vi "WW_GatherSpinParameter_V2.vi"(11 "路径":path) -> (0 "strFinishStepIndex":T1, 1 "strFinalSpinStepIndex":T2, 2 "strProgressStateIndex":T3, 3 "strPowerStateIndex":T5, 4 "EXCEL读取":string[][](array[string]), 5 "ms32ArrayLength":i32, 6 "strInitProgressStepIndex":T4)   [LabVIEW 2011]
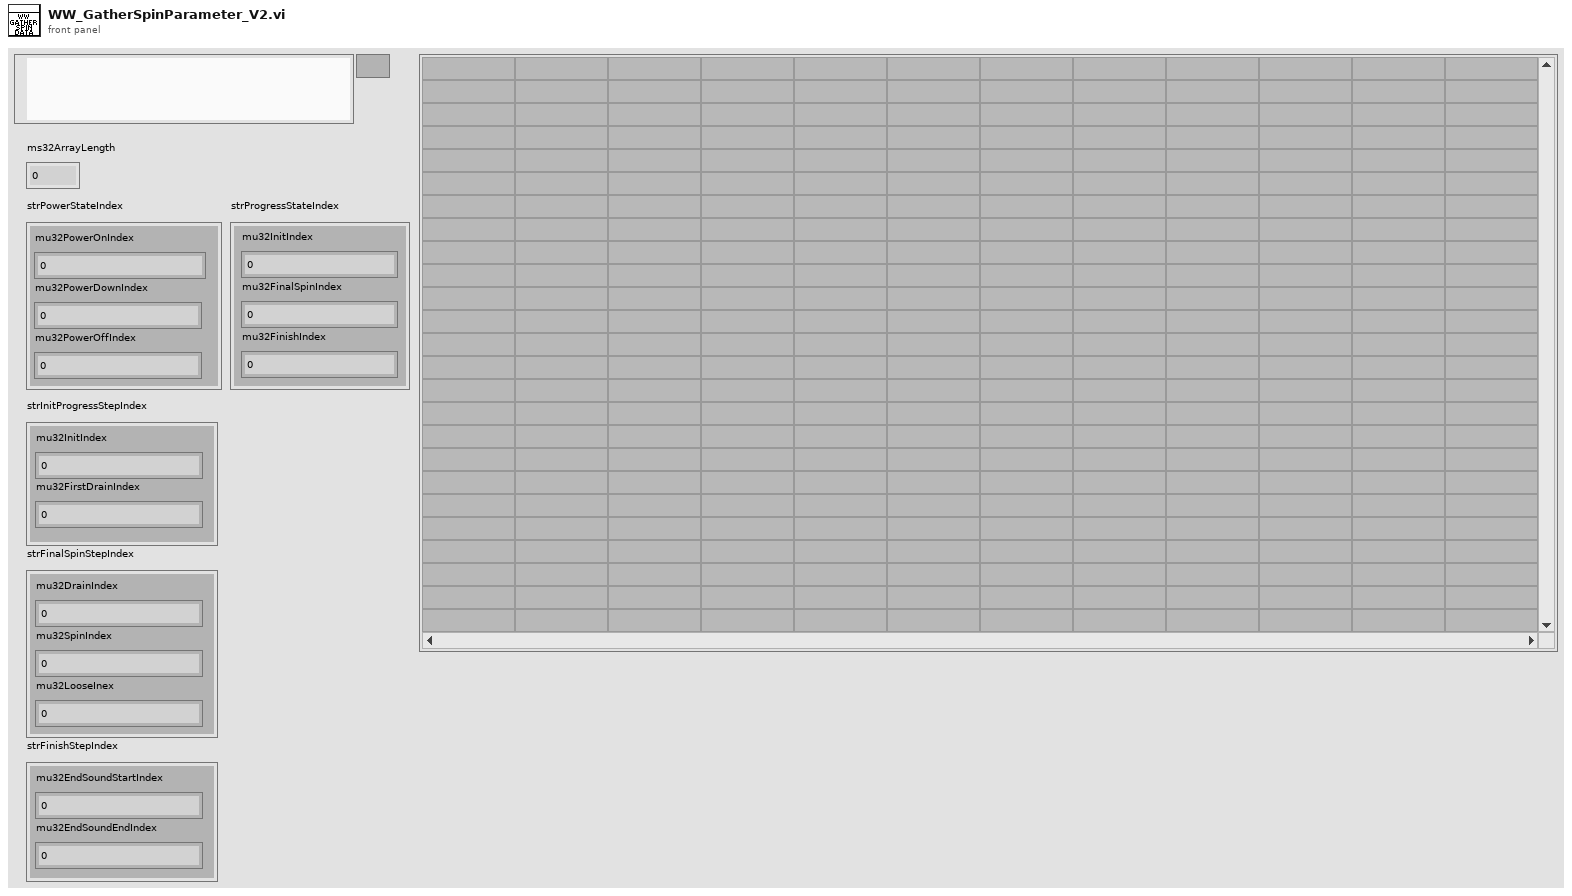
[diagram p1: front panel]
types:
  T1 = cluster{"mu32EndSoundStartIndex":u32, "mu32EndSoundEndIndex":u32}
  T2 = cluster{"mu32DrainIndex":u32, "mu32SpinIndex":u32, "mu32LooseInex":u32}
  T3 = cluster{"mu32InitIndex":u32, "mu32FinalSpinIndex":u32, "mu32FinishIndex":u32}
  T4 = cluster{"mu32InitIndex":u32, "mu32FirstDrainIndex":u32}
  T5 = cluster{"mu32PowerOnIndex":u32, "mu32PowerDownIndex":u32, "mu32PowerOffIndex":u32}
  T6 = enum16{"RealTime", "WaterLevel", "WaterTemp", "AirTemp", "IPMTemp", "MotorActualRPM", "MotorTargetRPM", "FanActualRPM", "MemsSensorA", "MemsSensorB", "MemsSensorC", "WaterThermistorADC", "TouchSensor", "LeakageSensor", "DCLink", "IsDoorOpen", "IsTimeShort", "Progress", "Step", "TotalRemainTime", "StepRemainTime", "WeightSensingLowData", "WeightSensingResult", "ColdValve", "HotValve", "PreValve", "WaterShotValve", "BleachValve", "DryValve", "SteamValve", "SoftenerValve", "FilterValve", "IsDoorLocked", "SSRCommon", "MainRelay", "ACTUATOR2", "WaterDrainer", "CirculationPump", "WaterHeater", "DryHeater", "SteamHeater", "MotorDriveDirection", "IsDoubleDoorOpen", "IsDoubleDoorLock", "RunStateID", "PowerStateID", "SoundID", "ErrorCode", "OptionData", "MainVersion", "SUBVersion", "InverterVersion"}
  T7 = enum16{"POWER_STATE_POWER_OFF", "POWER_STATE_POWER_UP_INIT", "POWER_STATE_POWER_UP_START", "POWER_STATE_POWER_UP_DONE", "POWER_STATE_POWER_ON", "POWER_STATE_POWER_DOWN", "POWER_STATE_POWER_OFF_FOR_OTN", "POWER_STATE_POWER_SLEEP_MODE"}
  T8 = enum16{"PROGRESS_INITIAL", "PROGRESS_RESERVE", "PROGRESS_PREWASH", "PROGRESS_WASH", "PROGRESS_RINSE", "PROGRESS_FINALSPIN", "PROGRESS_DRY", "PROGRESS_AIRWASH", "PROGRESS_FINISH", "PROGRESS_END", "PROGRESS_MAX"}
  T9 = enum16{"INIT_PROGRESS_INIT", "INIT_PROGRESS_FIRST_DRAIN_INITIAL", "INIT_PROGRESS_FIRST_DRAIN"}
  T10 = enum16{"FINALSPIN_INIT", "FINALSPIN_DRAIN", "FINALSPIN_SUDS_REDUCTION", "FINALSPIN_SPIN", "FINALSPIN_LOOSE", "FINALSPIN_END"}
  T11 = enum16{"FINISH_STEPORDER_COUNT_INFORMATION_SAVE", "FINISH_STEPORDER_ENDSOUND_PLAY", "FINISH_STEPORDER_UNLOCK_CHECK", "FINISH_STEPORDER_AGING_WAITTIME_CHECK", "FINISH_STEPORDER_AGING_WAITTING", "FINISH_STEPORDER_NOMAL_WAITTING", "FINISH_STEPORDER_DRUMLIGHT_CHECK", "FINISH_STEPORDER_CHECK_MOTOR_STOP", "FINISH_STEPORDER_CHILDLOCK_WAITTING", "FINISH_STEPORDER_CLOSE"}
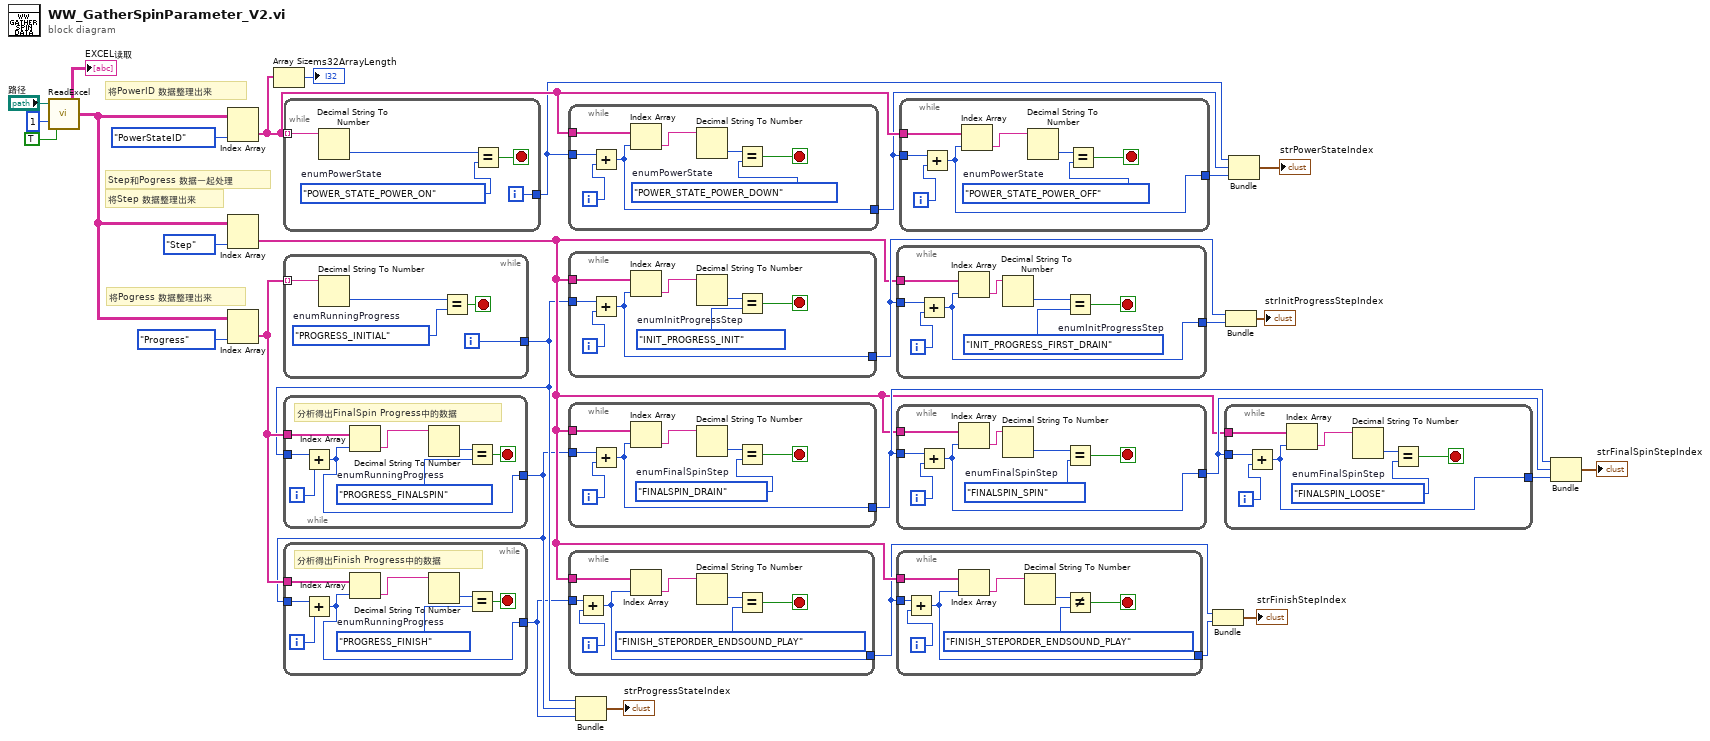
[diagram p0: block diagram]
diagram:
  # "Step和Pogress 数据一起处理"
  # "将Step 数据整理出来"
  # "将Pogress 数据整理出来"
  # "将PowerID 数据整理出来"
  n1 = call "ReadExcel.vi"("读出文本"=TRUE, "导出sheet位号"=i8 1, "路径"="路径") -> ("EXCEL读取"=w15:string[][])
  "EXCEL读取" <- w15
  n2 = Index Array(array=w15, index (col)=T6."PowerStateID" ("WW_ParameterData")) -> (element=w24:string[])  [unwired: 1 in]
  n3 = Index Array(array=w15, index (col)=T6."Step" ("WW_ParameterData")) -> (element=w8:string[])  [unwired: 1 in]
  n4 = Index Array(array=w15, index (col)=T6."Progress" ("WW_ParameterData")) -> (element=w9:string[])  [unwired: 1 in]
  n5 = Array Size(array=w24) -> (size(s)=→"ms32ArrayLength":i32)
  n6 = while {
    tunnel: w24 -> [w34] mode=indexing
    tunnel: [w30] -> w23
    i -> [w30]
    stop <- w31 stop-if-true
    w32 = T7."POWER_STATE_POWER_ON"  # enumPowerState
    n7 = Decimal String To Number(string=w34) -> (number=w33:i32)  [unwired: 2 in, 1 out]
    n8 = Equal?(x=w33, y=w32) -> (x = y?=w31:bool)
  }
  n9 = while {
    tunnel: w9 -> [w39] mode=indexing
    tunnel: [w36] -> w4
    i -> [w36]
    stop <- w37 stop-if-true
    w35 = T8."PROGRESS_INITIAL"  # enumRunningProgress
    n10 = Decimal String To Number(string=w39) -> (number=w38:i32)  [unwired: 2 in, 1 out]
    n11 = Equal?(x=w38, y=w35) -> (x = y?=w37:bool)
  }
  n12 = while {
    tunnel: w9 -> [w42]
    tunnel: w4 -> [w43]
    tunnel: [w40] -> w3
    i -> [w44]
    stop <- w46 stop-if-true
    w45 = T8."PROGRESS_FINALSPIN"  # enumRunningProgress
    # "分析得出FinalSpin Progress中的数据"
    n13 = Add(x=w43, y=w44) -> (x+y=w40:i32)
    n14 = Index Array(array=w42, index=w40) -> (element=w41:string)
    n15 = Decimal String To Number(string=w41) -> (number=w47:i32)  [unwired: 2 in, 1 out]
    n16 = Equal?(x=w47, y=w45) -> (x = y?=w46:bool)
  }
  n17 = while {
    tunnel: w9 -> [w50]
    tunnel: w3 -> [w51]
    tunnel: [w48] -> w2
    i -> [w52]
    stop <- w54 stop-if-true
    w53 = T8."PROGRESS_FINISH"  # enumRunningProgress
    # "分析得出Finish Progress中的数据"
    n18 = Add(x=w51, y=w52) -> (x+y=w48:i32)
    n19 = Index Array(array=w50, index=w48) -> (element=w49:string)
    n20 = Decimal String To Number(string=w49) -> (number=w55:i32)  [unwired: 2 in, 1 out]
    n21 = Equal?(x=w55, y=w53) -> (x = y?=w54:bool)
  }
  n22 = while {
    tunnel: w24 -> [w58]
    tunnel: w23 -> [w59]
    tunnel: [w56] -> w22
    i -> [w60]
    stop <- w61 stop-if-true
    w62 = T7."POWER_STATE_POWER_DOWN"  # enumPowerState
    n23 = Add(x=w59, y=w60) -> (x+y=w56:i32)
    n24 = Index Array(array=w58, index=w56) -> (element=w57:string)
    n25 = Decimal String To Number(string=w57) -> (number=w63:i32)  [unwired: 2 in, 1 out]
    n26 = Equal?(x=w63, y=w62) -> (x = y?=w61:bool)
  }
  n27 = while {
    tunnel: w8 -> [w67]
    tunnel: w4 -> [w68]
    tunnel: [w65] -> w18
    i -> [w69]
    stop <- w70 stop-if-true
    w64 = T9."INIT_PROGRESS_INIT"  # enumInitProgressStep
    n28 = Add(x=w68, y=w69) -> (x+y=w65:i32)
    n29 = Index Array(array=w67, index=w65) -> (element=w66:string)
    n30 = Decimal String To Number(string=w66) -> (number=w71:i32)  [unwired: 2 in, 1 out]
    n31 = Equal?(x=w71, y=w64) -> (x = y?=w70:bool)
  }
  n32 = while {
    tunnel: w8 -> [w75]
    tunnel: w3 -> [w76]
    tunnel: [w73] -> w13
    i -> [w77]
    stop <- w78 stop-if-true
    w72 = T10."FINALSPIN_DRAIN"  # enumFinalSpinStep
    n33 = Add(x=w76, y=w77) -> (x+y=w73:i32)
    n34 = Index Array(array=w75, index=w73) -> (element=w74:string)
    n35 = Decimal String To Number(string=w74) -> (number=w79:i32)  [unwired: 2 in, 1 out]
    n36 = Equal?(x=w79, y=w72) -> (x = y?=w78:bool)
  }
  n37 = while {
    tunnel: w8 -> [w83]
    tunnel: w2 -> [w84]
    tunnel: [w81] -> w7
    i -> [w85]
    stop <- w86 stop-if-true
    n38 = Add(x=w84, y=w85) -> (x+y=w81:i32)
    n39 = Index Array(array=w83, index=w81) -> (element=w82:string)
    n40 = Decimal String To Number(string=w82) -> (number=w87:i32)  [unwired: 2 in, 1 out]
    n41 = Equal?(x=w87, y=T11."FINISH_STEPORDER_ENDSOUND_PLAY" ("enumFinishStep")) -> (x = y?=w86:bool)
  }
  n42 = Bundle(w4, w3, w2) -> (→"strProgressStateIndex":cluster{i32, i32, i32})  [unwired: 1 in]
  n43 = while {
    tunnel: w8 -> [w91]
    tunnel: w18 -> [w92]
    tunnel: [w89] -> w17
    i -> [w93]
    stop <- w94 stop-if-true
    w88 = T9."INIT_PROGRESS_FIRST_DRAIN"  # enumInitProgressStep
    n44 = Add(x=w92, y=w93) -> (x+y=w89:i32)
    n45 = Index Array(array=w91, index=w89) -> (element=w90:string)
    n46 = Decimal String To Number(string=w90) -> (number=w95:i32)  [unwired: 2 in, 1 out]
    n47 = Equal?(x=w95, y=w88) -> (x = y?=w94:bool)
  }
  n48 = while {
    tunnel: w8 -> [w99]
    tunnel: w13 -> [w100]
    tunnel: [w97] -> w12
    i -> [w101]
    stop <- w102 stop-if-true
    w96 = T10."FINALSPIN_SPIN"  # enumFinalSpinStep
    n49 = Add(x=w100, y=w101) -> (x+y=w97:i32)
    n50 = Index Array(array=w99, index=w97) -> (element=w98:string)
    n51 = Decimal String To Number(string=w98) -> (number=w103:i32)  [unwired: 2 in, 1 out]
    n52 = Equal?(x=w103, y=w96) -> (x = y?=w102:bool)
  }
  n53 = while {
    tunnel: w8 -> [w107]
    tunnel: w7 -> [w108]
    tunnel: [w105] -> w6
    i -> [w109]
    stop <- w110 stop-if-true
    n54 = Add(x=w108, y=w109) -> (x+y=w105:i32)
    n55 = Index Array(array=w107, index=w105) -> (element=w106:string)
    n56 = Decimal String To Number(string=w106) -> (number=w111:i32)  [unwired: 2 in, 1 out]
    n57 = Not Equal?(x=w111, y=T11."FINISH_STEPORDER_ENDSOUND_PLAY" ("enumFinishStep")) -> (x != y?=w110:bool)
  }
  n58 = while {
    tunnel: w24 -> [w114]
    tunnel: w22 -> [w115]
    tunnel: [w112] -> w21
    i -> [w116]
    stop <- w117 stop-if-true
    w118 = T7."POWER_STATE_POWER_OFF"  # enumPowerState
    n59 = Add(x=w115, y=w116) -> (x+y=w112:i32)
    n60 = Index Array(array=w114, index=w112) -> (element=w113:string)
    n61 = Decimal String To Number(string=w113) -> (number=w119:i32)  [unwired: 2 in, 1 out]
    n62 = Equal?(x=w119, y=w118) -> (x = y?=w117:bool)
  }
  n63 = Bundle(w7, w6) -> (→"strFinishStepIndex":cluster{i32, i32})  [unwired: 1 in]
  n64 = while {
    tunnel: w8 -> [w123]
    tunnel: w12 -> [w124]
    tunnel: [w120] -> w11
    i -> [w125]
    stop <- w126 stop-if-true
    w121 = T10."FINALSPIN_LOOSE"  # enumFinalSpinStep
    n65 = Add(x=w124, y=w125) -> (x+y=w120:i32)
    n66 = Index Array(array=w123, index=w120) -> (element=w122:string)
    n67 = Decimal String To Number(string=w122) -> (number=w127:i32)  [unwired: 2 in, 1 out]
    n68 = Equal?(x=w127, y=w121) -> (x = y?=w126:bool)
  }
  n69 = Bundle(w18, w17) -> (→"strInitProgressStepIndex":cluster{i32, i32})  [unwired: 1 in]
  n70 = Bundle(w23, w22, w21) -> (→"strPowerStateIndex":cluster{i32, i32, i32})  [unwired: 1 in]
  n71 = Bundle(w13, w12, w11) -> (→"strFinalSpinStepIndex":cluster{i32, i32, i32})  [unwired: 1 in]
